vi "簇.vi"() -> ()   [LabVIEW 2015]
panel:
  out "Slide":dbl(slide) scale=0.0..10.0
  out "String":string
  out "Boolean":bool
  out "Numeric":dbl
  out "Cluster 4":T1 {"Slide" scale=0.0..10.0}
  in  "Cluster 3":T1 {"Slide" scale=0.0..10.0}
  out "Cluster 2":T2
  out "Array 2":bool[](array[boolean])
  in  "Cluster":T2
  out "Array":bool[](array[boolean])
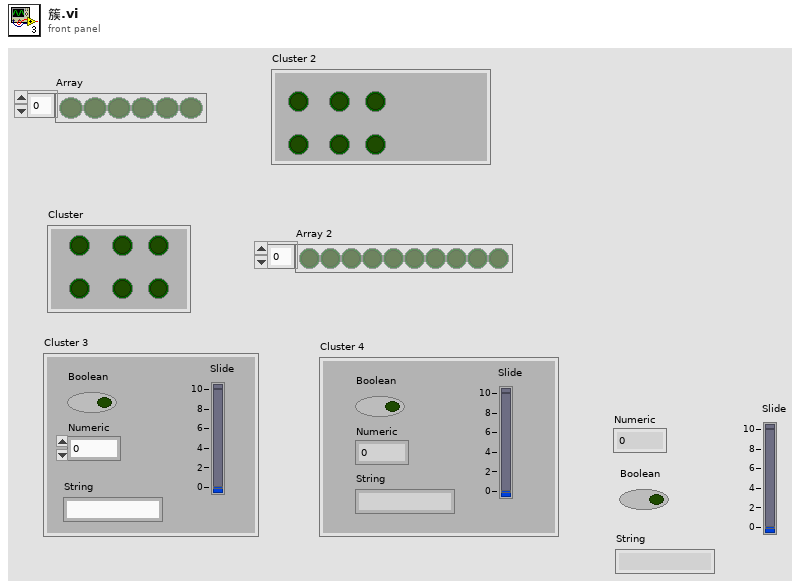
[diagram p1: front panel]
types:
  T1 = cluster{"Boolean":bool, "Numeric":dbl, "String":string, "Slide":dbl}
  T2 = cluster{"Boolean":bool, "Boolean 2":bool, "Boolean 3":bool, "Boolean 4":bool, "Boolean 5":bool, "Boolean 6":bool}
  T3 = cluster{"[0]":bool, "[1]":bool, "[2]":bool, "[3]":bool, "[4]":bool, "[5]":bool}
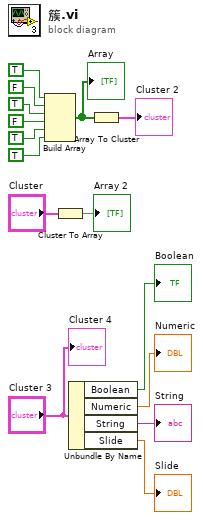
[diagram p0: block diagram]
diagram:
  n1 = Build Array(TRUE, FALSE, TRUE, FALSE, TRUE, TRUE) -> (w7:bool[])
  "Array" <- w7
  n2 = Cluster To Array(cluster="Cluster") -> (array=→"Array 2":bool[])
  n3 = Unbundle By Name("Cluster 3") -> ("Boolean"=→"Boolean":bool, "Numeric"=→"Numeric":dbl, "String"=→"String":string, "Slide"=→"Slide":dbl)
  n4 = Array To Cluster(array=w7) -> (cluster=→"Cluster 2":T3)
  "Cluster 4" <- "Cluster 3"
